vi "Set Waypoint Type BG.vi"(8 "Error In":errorcluster, 10 "Waypoint Type Ref":refnum<vi>, 11 "Waypoint Type":T1) -> (0 "Error Out":errorcluster)   [LabVIEW 2014]
uses:
  Missions/Controls/Waypoint Type.ctl
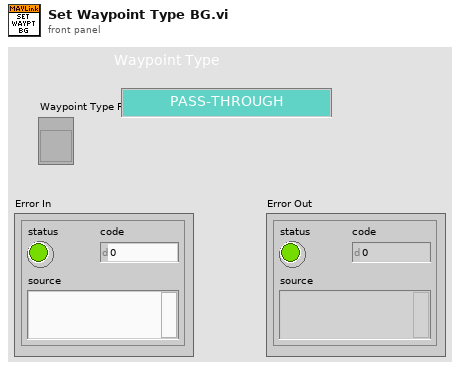
[diagram p1: front panel]
types:
  T1 = typedef "Waypoint Type.ctl" = enum16{"PASS-THROUGH", "INSPECT", "CIRCUMNAVIGATE"}
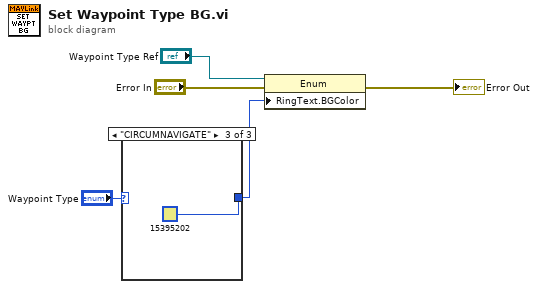
[diagram p0: block diagram]
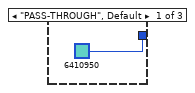
[diagram p2: hidden frame]
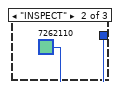
[diagram p3: hidden frame]
diagram:
  n1 = case shown="\"CIRCUMNAVIGATE\"" "Waypoint Type" {
    tunnel: [u32 6410950 u32 7262110 u32 15395202] -> w1
    frame "PASS-THROUGH", Default {
    }
    frame "INSPECT" {
    }
    frame "CIRCUMNAVIGATE" {
    }
  }
  n2 = property class="Enum"(reference="Waypoint Type Ref", error in="Error In", "RingText.BGColor"=w1) -> (error out=→"Error Out":errorcluster)  [unwired: 1 out]
